vi "Counter Mode.vi"(7 "Read Value? (F)":bool, 8 "error in (no error)":errorcluster, 10 "Counter Mode (A,B for T preset)":T1, 11 "VISA resource name":refnum<visa-resource-name>) -> (0 "error out":errorcluster, 2 "Counter Mode":T1, 3 "VISA resource name out":refnum<visa-resource-name>)   [LabVIEW 2013, in "SRS SR400.lvlib"]
doc: "<B>CM { j }</B>\n\nIf j is included, the CM command sets the counting mode. If j is absent, the counting mode is returned.\n\n<B>j</B> <B>Counting Mode</B>\n0 A,B FOR T PRESET\n1 A-B FOR T PRESET\n2 A+B FOR T PRESET\n3 A FOR B PRESET\n\nSetting the counter mode also performs a counter reset."
uses:
  <instrlib>/SRS SR400/SRS SR400.lvlib
  <instrlib>/SRS SR400/Public/Typedefs/Counter Mode.ctl
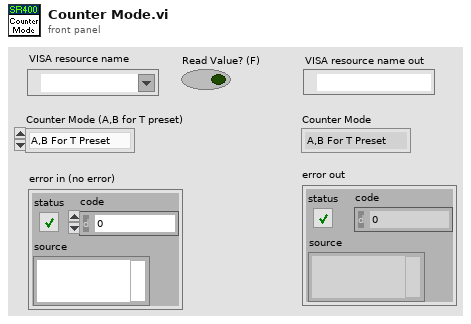
[diagram p1: front panel]
types:
  T1 = typedef "SRS SR400.lvlib/Counter Mode.ctl" = enum16{"A,B For T Preset", "A-B For T Preset", "A+B For T Preset", "A For B Preset"}
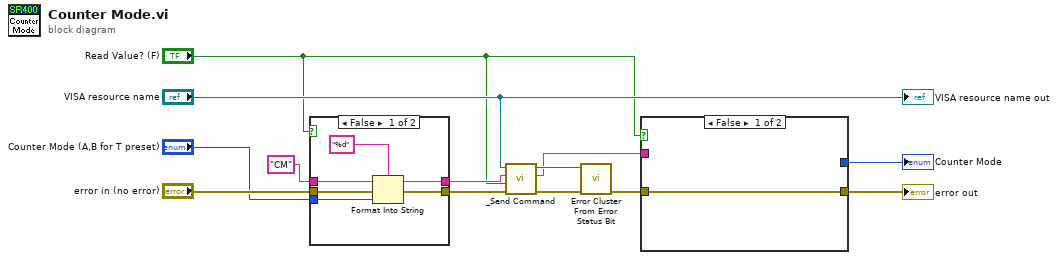
[diagram p0: block diagram]
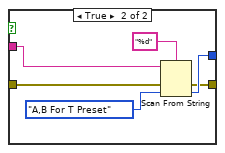
[diagram p2: hidden frame]
diagram:
  n1 = case shown="False" "Read Value? (F)" {
    tunnel: "error in (no error)" -> [w19 w21]
    tunnel: "Counter Mode (A,B for T preset)" -> [w17 _]
    tunnel: [w16 w20] -> w11
    tunnel: [w15 w21] -> w10
    tunnel: "CM" ("command") -> [w14 w20]
    frame False {
      n2 = Format Into String(format string="%d", initial string=w14, error in=w19, w17) -> (resulting string=w16:string, error out=w15:errorcluster)
    }
    frame True {
    }
  }
  n3 = call <instrlib>:"_Send Command.vi"("error in (no error)"=w10, "Read Value? (F)"="Read Value? (F)", "Command"=w11, "VISA resource name"="VISA resource name") -> ("error out"=w8:errorcluster, "Response"=w1:string, "VISA resource name out"=w9:refnum<visa-resource-name>)  [unwired: 5 out]
  n4 = call <instrlib>:"Error Cluster From Error Status Bit.vi"("error in (no error)"=w8, "VISA resource name"=w9) -> ("error out"=w5:errorcluster)  [unwired: 8 in, 1 out]
  n5 = case shown="False" "Read Value? (F)" {
    tunnel: w5 -> [w22 w28]
    tunnel: [_ w25] -> w4
    tunnel: [w22 w24] -> w3
    tunnel: w1 -> [_ w23]
    frame False {
    }
    frame True {
      n6 = Scan From String(format string="%d", input string=w23, error in=w28, default 1=Counter_Mode."A,B For T Preset" ("Counter Mode (A,B for T preset)")) -> (error out=w24:errorcluster, output 1=w25:T1)  [unwired: 1 in, 2 out]
    }
  }
  "error out" <- w3
  "Counter Mode" <- w4
  "VISA resource name out" <- "VISA resource name"
